vi "Draw Vector Polar Plot.vi"(7 "Pcture Refnum In":refnum<vi>, 8 "Error In (no Error) In":errorcluster, 9 "Display State In":T1 caption="State", 10 "In":cluster{dbl, dbl}[](array[cluster]), 11 "Plot In":picture) -> (0 "Error Out":errorcluster, 3 "Plot Out":picture)   [LabVIEW 2012, in "Vector Function Generator.xctl"]
doc: "Takes either R,theta or X,Y data points and the XControl's current state and plots the appropriate data"
uses:
  Vector Function Generator.xctl
  Vector State.ctl
  <vilib>/picture/cartesn2.llb/XY Plot Type.ctl
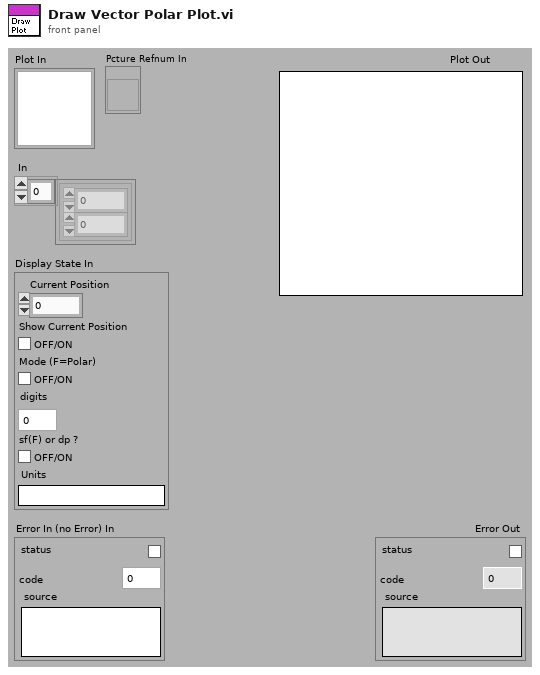
[diagram p1: front panel]
types:
  T1 = typedef "Vector Function Generator.xctl/Vector State.ctl" = cluster{"Current Position":i32, "Show Current Position":bool, "Mode (F=Polar)":bool, "digits":i32, "sf(F) or dp ?":bool, "Units":string}
  T2 = cluster{"maximum":dbl, "minimum":dbl, "clip to min":bool, "log?(F)":bool, "grid color":u32, "plot color":u32, "fmt and prec":cluster{"format":enum8{"Decimal", "Scientific", "Engineering", "Binary", "Octal", "Hex"}, "precision":u8}, "visible section":u16}
  T3 = cluster{"x minimum":dbl, "x maximum":dbl, "x log?":bool, "x precision":u8, "x format":enum8{"Decimal", "Scientific", "Engineering", "Binary", "Octal", "Hex"}, "y minimum":dbl, "y maximum":dbl, "y log?":bool, "y precision":u8, "y format":enum8{"Decimal", "Scientific", "Engineering", "Binary", "Octal", "Hex"}}
  T4 = typedef "XY Plot Type.ctl" = enum16{"points", "squares", "circles", "connected points", "connected squares", "connected circles", "comb plot", "sized scatter plot", "sized-colored scatter plot", "min-max lines"}
  T5 = cluster{"plot color":u32, "XY plot type":T4, "baseline":dbl}
  T6 = cluster{"line color":u32, "text color":u32, "tick length(3)":i16, "crossing axes":bool, "visible grid?":bool}
  T7 = cluster{"plot color":u32, "XY plot type":T4, "baseline":dbl}[]
  T8 = typedef "LVBoundsTypeDef.ctl" = cluster{"Width":u32, "Height":u32}
  T9 = cluster{"pixel center":cluster{"x":i16, "y":i16}, "scale factors":cluster{"a":dbl, "b":dbl, "log?":bool}, "grid color":u32, "start angle":dbl, "end angle":dbl, "tick length":i16, "pixel radius":i32}
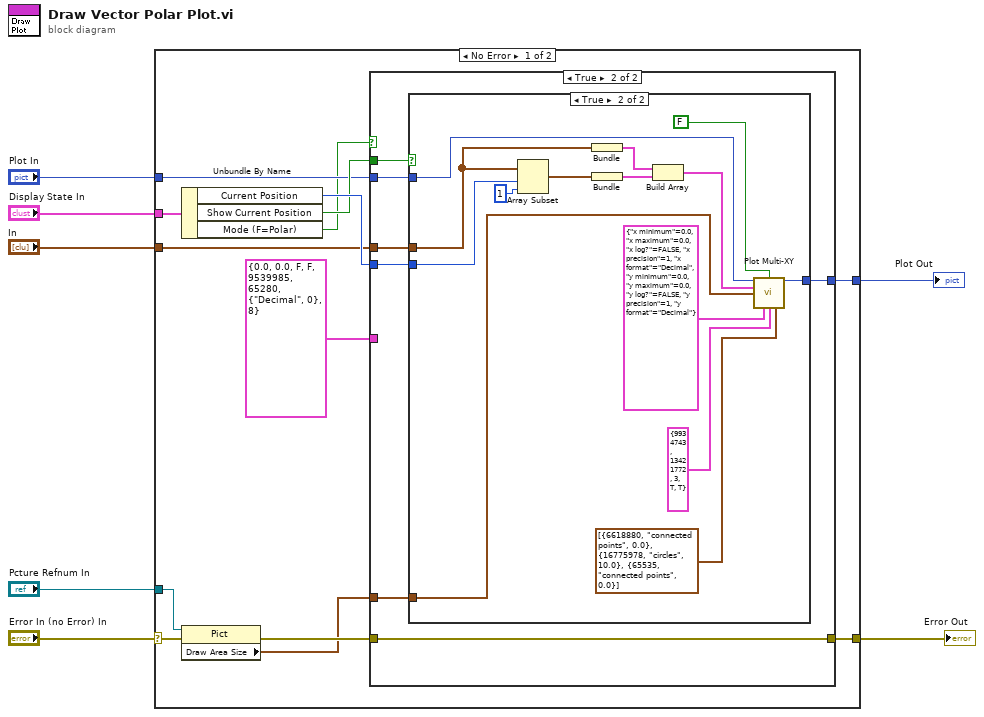
[diagram p0: block diagram]
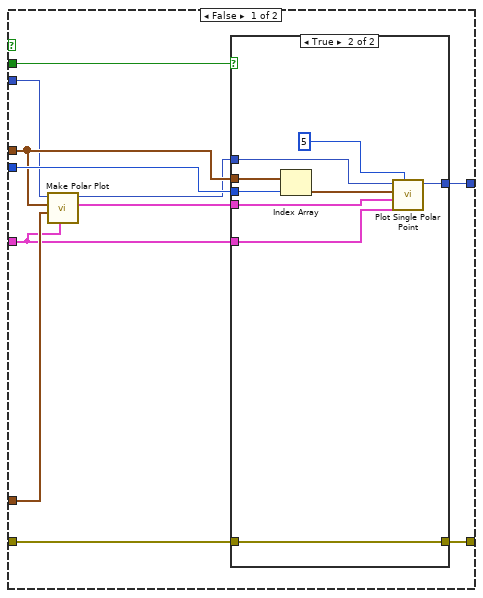
[diagram p2: hidden frame]
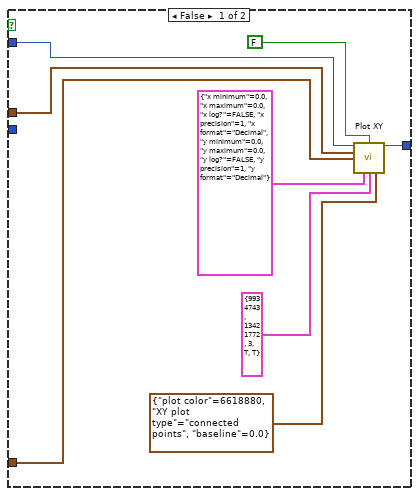
[diagram p4: hidden frame]
diagram:
  n1 = case shown="No Error" "Error In (no Error) In" {
    selector: "Error In (no Error) In" -> [w10 w72]
    tunnel: [w20 _] -> w7
    tunnel: "In" -> [w18 _]
    tunnel: "Display State In" -> [w16 _]
    tunnel: [w15 w72] -> w4
    tunnel: "Plot In" -> [w14 _]
    tunnel: "Pcture Refnum In" -> [w11 _]
    frame No Error {
      n2 = Unbundle By Name(w16) -> ("Current Position"=w19:i32, "Show Current Position"=w17:bool, "Mode (F=Polar)"=w13:bool)
      n3 = property class="Pict"(reference=w11, error in=w10) -> (error out=w9:errorcluster, "Draw Area Size"=w8:T8)  [unwired: 1 out]
      n4 = case shown="True" w13 {
        tunnel: [w31 w47] -> w20
        tunnel: w19 -> [w29 w43]
        tunnel: w18 -> [w28 w48]
        tunnel: w17 -> [w26 w44]
        tunnel: w9 -> [w25 w46]
        tunnel: [w24 w46] -> w15
        tunnel: w14 -> [w23 w49]
        tunnel: w8 -> [w22 w45]
        tunnel: T2 {"maximum"=0.0, "minimum"=0.0, "clip to min"=FALSE, "log?(F)"=FALSE, "grid color"=9539985, "plot color"=65280, "fmt and prec"={"format"=enum."Decimal", "precision"=0}, "visible section"=8} ("polar attributes") -> [w21 _]
        frame False {
          n5 = call "Make Polar Plot.vi"("polar attributes"=w21, "dimensions (w,h)"=w22, "data array [mag, phase (deg)]"=w28, "picture"=w23) -> ("grid measurements"=w30:T9, "new picture"=w27:picture)  [unwired: 6 out]
          n6 = case shown="True" w26 {
            tunnel: w27 -> [w32 w39]
            tunnel: w28 -> [_ w42]
            tunnel: w29 -> [_ w41]
            tunnel: w21 -> [_ w37]
            tunnel: w30 -> [_ w36]
            tunnel: [w32 w35] -> w31
            tunnel: [w33 w34] -> w24
            tunnel: w25 -> [w33 w34]
            frame False {
            }
            frame True {
              n7 = Index Array(array=w42, index=w41) -> (element=w40:cluster{dbl, dbl})
              n8 = call "Plot Single Polar Point.vi"("Size"=i16 5, "polar attributes"=w37, "grid measurements"=w36, "Polar Point"=w40, "picture"=w39) -> ("new picture"=w35:picture)  [unwired: 1 in, 5 out]
            }
          }
        }
        frame True {
          n9 = case shown="True" w44 {
            tunnel: w49 -> [w57 w71]
            tunnel: w48 -> [w56 w62]
            tunnel: [w55 w70] -> w47
            tunnel: w45 -> [w54 w69]
            tunnel: w43 -> [_ w61]
            frame False {
              n10 = call "Plot XY.vi"("picture"=w57, "Draw Axes"=FALSE, "data"=w56, "dimensions (w,h)"=w54, "cartesian axis attributes"=T3 {"x minimum"=0.0, "x maximum"=0.0, "x log?"=FALSE, "x precision"=1, "x format"=enum."Decimal", "y minimum"=0.0, "y maximum"=0.0, "y log?"=FALSE, "y precision"=1, "y format"=enum."Decimal"}, "cartesian grid cosmetics"=T6 {"line color"=9934743, "text color"=13421772, "tick length(3)"=3, "crossing axes"=TRUE, "visible grid?"=TRUE}, "XY plot cosmetics"=T5 {"plot color"=6618880, "XY plot type"=enum."connected points", "baseline"=0.0}) -> ("new picture"=w55:picture)  [unwired: 1 in, 7 out]
            }
            frame True {
              n11 = Array Subset(array=w62, index=w61, length=1) -> (w59:cluster{dbl, dbl}[])
              n12 = Bundle("In"=w62) -> (w65:cluster{" In":cluster{dbl, dbl}[]})  [unwired: 1 in]
              n13 = Bundle(w59) -> (w63:cluster{cluster{dbl, dbl}[]})  [unwired: 1 in]
              n14 = Build Array(w65, w63) -> (w64:cluster{" In":cluster{dbl, dbl}[]}[])
              n15 = call "Plot Multi-XY.vi"("picture"=w71, "Draw Axes"=FALSE, "data"=w64, "dimensions (w,h)"=w69, "cartesian axis attributes"=T3 {"x minimum"=0.0, "x maximum"=0.0, "x log?"=FALSE, "x precision"=1, "x format"=enum."Decimal", "y minimum"=0.0, "y maximum"=0.0, "y log?"=FALSE, "y precision"=1, "y format"=enum."Decimal"}, "cartesian grid cosmetics"=T6 {"line color"=9934743, "text color"=13421772, "tick length(3)"=3, "crossing axes"=TRUE, "visible grid?"=TRUE}, "XY plot cosmetics"=T7 [{"plot color"=6618880, "XY plot type"=enum."connected points", "baseline"=0.0}, {"plot color"=16775978, "XY plot type"=enum."circles", "baseline"=10.0}, {"plot color"=65535, "XY plot type"=enum."connected points", "baseline"=0.0}]) -> ("new picture"=w70:picture)  [unwired: 1 in, 7 out]
            }
          }
        }
      }
    }
    frame Error {
    }
  }
  "Plot Out" <- w7
  "Error Out" <- w4
